vi "LS218_READ_ETAT_8VOIES.vi"(8 "entrée d'erreur":errorcluster, 10 "Voies de mesures":T2(array[cluster]), 11 "Refnum VISA en entrée":refnum<visa-resource-name>) -> (0 "sortie d'erreur":errorcluster, 2 "Tableau":T1(array[cluster]), 3 "Nom de ressource VISA en sortie":refnum<visa-resource-name>)   [LabVIEW 2016]
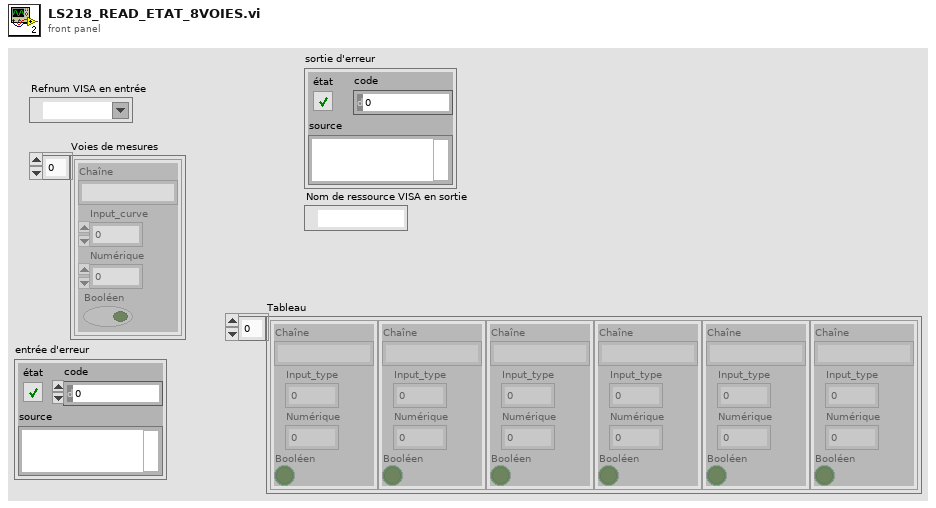
[diagram p1: front panel]
types:
  T1 = cluster{"Chaîne":string, "Input_type":u16, "Numérique":dbl, "Booléen":bool}[]
  T2 = cluster{"Chaîne":string, "Input_curve":u16, "Numérique":dbl, "Booléen":bool}[]
  T3 = cluster{"Chaîne":string, "Input_curve":u16, "Numérique":dbl, "Booléen":bool}
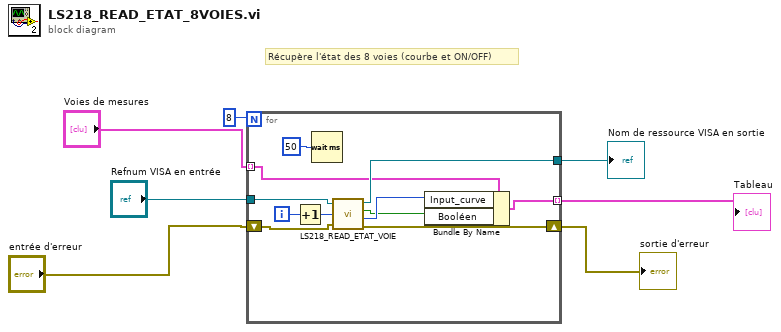
[diagram p0: block diagram]
diagram:
  # "Récupère l'état des 8 voies (courbe et ON/OFF)"
  n1 = for {
    N: 8 -> [_]
    tunnel: "Refnum VISA en entrée" -> [w14]
    shift-right: [w13] -> w5
    shift-left: "entrée d'erreur" -> [w16]
    tunnel: "Voies de mesures" -> [w11] mode=indexing
    tunnel: [w8] -> w3 mode=indexing
    tunnel: [w12] -> w4
    i -> [w17]
    n2 = Increment(x=w17) -> (x+1=w15:i32)
    n3 = Wait (ms)(milliseconds to wait=u32 50 ("attente (ms)")) -> ()  [unwired: 1 out]
    n4 = call "LS218_READ_ETAT_VOIE.vi"("Refnum VISA en entrée"=w14, "numéro voie"=w15, "entrée d'erreur (pas d'erreur)"=w16) -> ("Nom de ressource VISA en sortie"=w12:refnum<visa-resource-name>, "Input_ON"=w9:bool, "Input_curve"=w10:i32, "sortie d'erreur"=w13:errorcluster)
    n5 = Bundle By Name(cluster=w11, "Input_curve"=w10, "Booléen"=w9) -> (w8:T3)
  }
  "sortie d'erreur" <- w5
  "Nom de ressource VISA en sortie" <- w4
  "Tableau" <- w3
